vi "Meas Result Remove Readings.vi"(7 "ids of selected":i32[](array[numeric]), 8 "error in":errorcluster, 9 "sweep spot index":u16, 10 "phase index":u16, 11 "result":T1) -> (0 "error out":errorcluster, 3 "result out":T1)   [LabVIEW 2013]
doc: "Removes selected readings from result data."
uses:
  Meas Results.ctl
  bridge/Bridge Frequency Readings Data.ctl
  drivers/TWM client/Meas Proc QWTB Spectrum Data.ctl
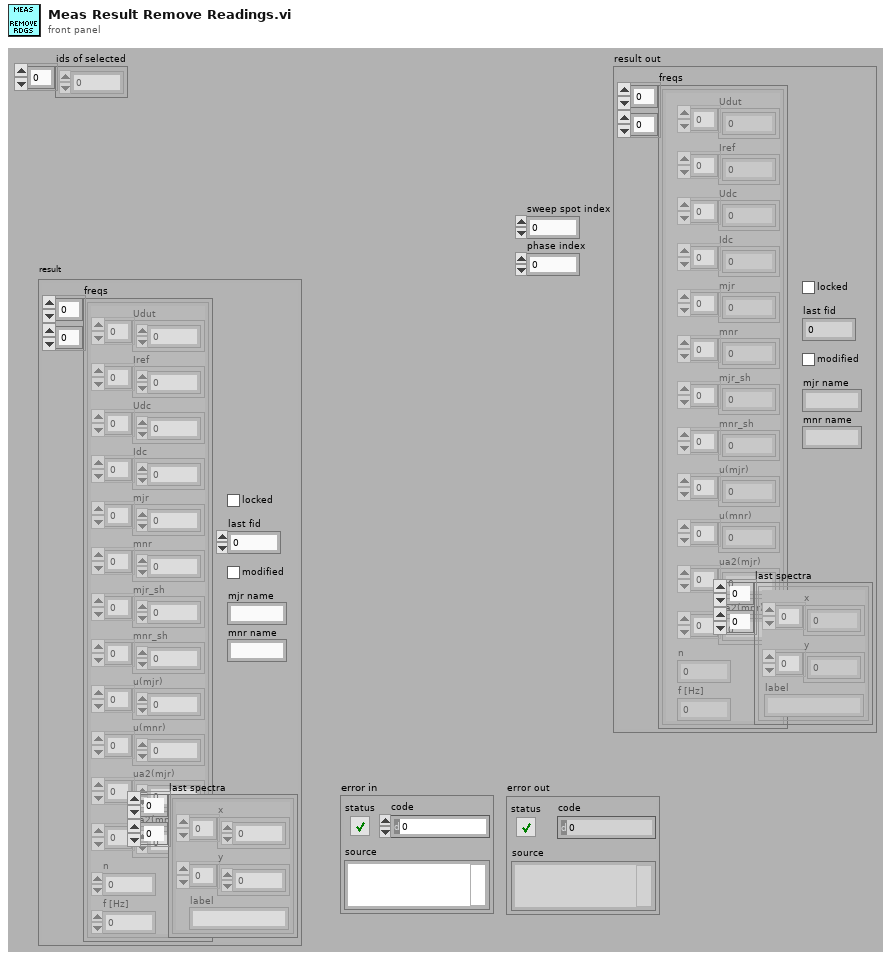
[diagram p1: front panel]
types:
  T1 = typedef "Meas Results.ctl" = cluster{"freqs":T2[][], "locked":bool, "last fid":i32, "modified":bool, "mjr name":string, "mnr name":string, "last spectra":T3[][]}
  T2 = typedef "Bridge Frequency Readings Data.ctl" = cluster{"Udut":dbl[], "Iref":dbl[], "Udc":dbl[], "Idc":dbl[], "mjr":dbl[], "mnr":dbl[], "mjr_sh":dbl[], "mnr_sh":dbl[], "u(mjr)":dbl[], "u(mnr)":dbl[], "ua2(mjr)":dbl[], "ua2(mnr)":dbl[], "n":i32, "f [Hz]":dbl}
  T3 = typedef "Meas Proc QWTB Spectrum Data.ctl" = cluster{"x":sgl[], "y":sgl[], "label":string}
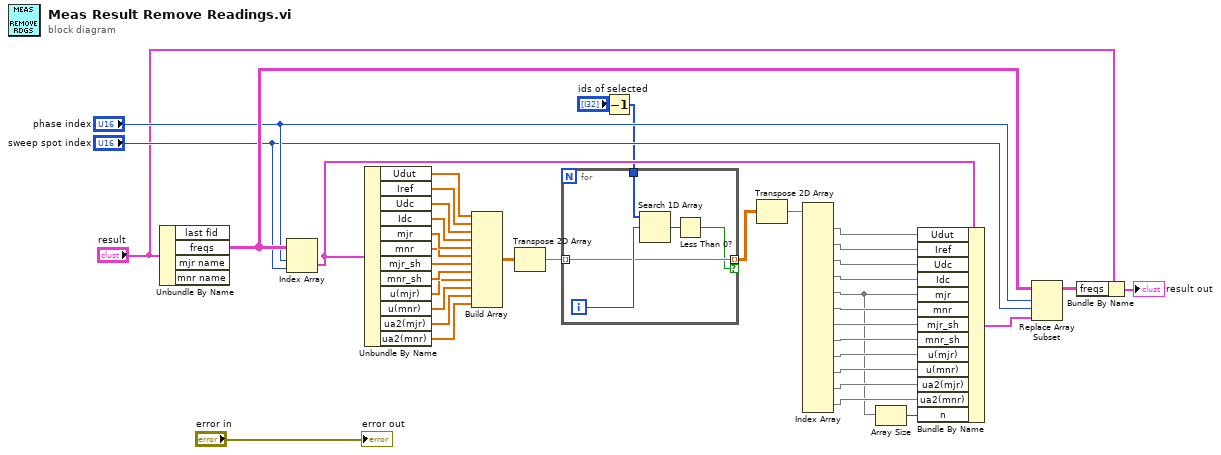
[diagram p0: block diagram]
diagram:
  n1 = Unbundle By Name("result") -> ("freqs"=w11:T2[][])  [unwired: 3 out]
  n2 = Index Array(array=w11, index (row)="phase index", index (col)="sweep spot index") -> (element=w23:T2)
  n3 = Unbundle By Name(w23) -> ("Udut"=w40:dbl[], "Iref"=w39:dbl[], "Udc"=w38:dbl[], "Idc"=w37:dbl[], "mjr"=w36:dbl[], "mnr"=w35:dbl[], "mjr_sh"=w34:dbl[], "mnr_sh"=w33:dbl[], "u(mjr)"=w32:dbl[], "u(mnr)"=w31:dbl[], "ua2(mjr)"=w30:dbl[], "ua2(mnr)"=w29:dbl[])
  n4 = Build Array(w40, w39, w38, w37, w36, w35, w34, w33, w32, w31, w30, w29) -> (w28:dbl[][])
  n5 = Transpose 2D Array(2D array=w28) -> (transposed array=w27:dbl[][])
  n6 = Decrement(x="ids of selected") -> (x-1=w1:i32[])
  n7 = for {
    tunnel: w27 -> [w43] mode=indexing
    tunnel: w1 -> [w45]
    tunnel: [w43] -> w25 mode=indexing if=w41
    i -> [w44]
    n8 = Search 1D Array(1D array=w45, element=w44) -> (index of element=w42:i32)  [unwired: 1 in]
    n9 = Less Than 0?(x=w42) -> (x < 0?=w41:bool)
  }
  n10 = Transpose 2D Array(2D array=w25) -> (transposed array=w24:dbl[][])
  n11 = Index Array(array=w24) -> (element #1=w22:dbl[], element #2=w21:dbl[], element #3=w20:dbl[], element #4=w19:dbl[], element #5=w6:dbl[], element #6=w18:dbl[], element #7=w17:dbl[], element #8=w16:dbl[], element #9=w15:dbl[], element #10=w14:dbl[], element #11=w13:dbl[], element #12=w7:dbl[])  [unwired: 24 in]
  n12 = Array Size(array=w6) -> (size(s)=w8:i32)
  n13 = Bundle By Name(cluster=w23, "Udut"=w22, "Iref"=w21, "Udc"=w20, "Idc"=w19, "mjr"=w6, "mnr"=w18, "mjr_sh"=w17, "mnr_sh"=w16, "u(mjr)"=w15, "u(mnr)"=w14, "ua2(mjr)"=w13, "ua2(mnr)"=w7, "n"=w8) -> (w12:T2)
  n14 = Replace Array Subset(array=w11, new element=w12, index (row)="phase index", index (col)="sweep spot index") -> (w4:T2[][])
  n15 = Bundle By Name(cluster="result", "freqs"=w4) -> (→"result out":T1)
  "error out" <- "error in"
